vi "Set XRT-U State.vi"(8 "error in (no error)":errorcluster, 11 "Inst.Xeryon-Rotator in":refnum<class "Inst.Xeryon-Rotator.lvclass">) -> (0 "error out":errorcluster, 3 "Inst.Xeryon-Rotator out":refnum<class "Inst.Xeryon-Rotator.lvclass">)   [LabVIEW 2019, in "Inst.Xeryon-Rotator.lvclass"]
uses:
  Inst.Xeryon-Rotator.lvclass
  drivers/Class/Controller/Controller.lvclass
panel:
  in  "Scan State":enum16{"Scan Left", "Stop", "Scan Right"}(ring)
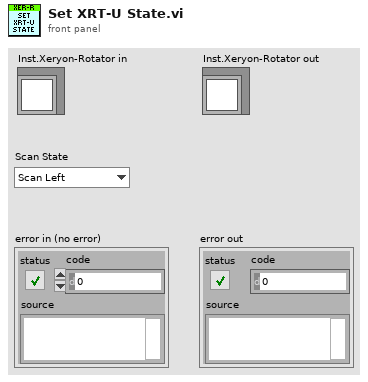
[diagram p1: front panel]
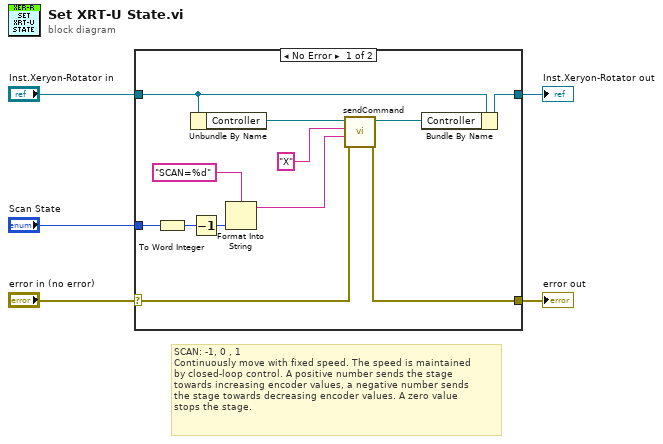
[diagram p0: block diagram]
diagram:
  # "SCAN: -1, 0 , 1\nContinuously move with fixed speed. The speed is maintained\nby closed-loop control. A positive number sends the stage\ntowards increasing encoder values, a negative number sends\nthe stage towards decreasing encoder values. A zero value\nstops the stage."
  n1 = case shown="No Error" "error in (no error)" {
    selector: "error in (no error)" -> [w13 w19]
    tunnel: "Inst.Xeryon-Rotator in" -> [w16 w18]
    tunnel: [w12 w19] -> w3
    tunnel: "Scan State" -> [w11 _]
    tunnel: [w6 w18] -> w1
    frame No Error {
      n2 = To Word Integer(number=w11) -> (16bit integer=w10:i16)
      n3 = Unbundle By Name(w16) -> ("Controller"=w17:refnum<class "Controller.lvclass">)
      n4 = Decrement(x=w10) -> (x-1=w9:i16)
      n5 = Format Into String(format string="SCAN=%d", w9) -> (resulting string=w7:string)  [unwired: 2 in, 1 out]
      n6 = call-dynamic "sendCommand.vi"("error in (no error)"=w13, "Command"=w7, "Axis Letter"="X", "Controller in"=w17) -> ("error out"=w12:errorcluster, "Controller out"=w14:refnum<class "Controller.lvclass">)  [unwired: 6 in]
      n7 = Bundle By Name(cluster=w16, "Controller"=w14) -> (w6:refnum<class "Inst.Xeryon-Rotator.lvclass">)
    }
    frame Error {
    }
  }
  "Inst.Xeryon-Rotator out" <- w1
  "error out" <- w3
